vi "高低位调试.vi"() -> ()   [LabVIEW 2016]
uses:
  <vilib>/Plasmionique/MB Master/MB_Master_Serial/MB_Master_Serial.lvclass
  C:/Program Files (x86)/National Instruments/LabVIEW 2016/vi.lib/Plasmionique/MB Master/MB_Master/MB_Master.lvclass
  <vilib>/Plasmionique/MB Master/MB Master.lvlib
panel:
  out "data":u16[](array[numeric]) format="%04xH"
  out "测量数据区":T1
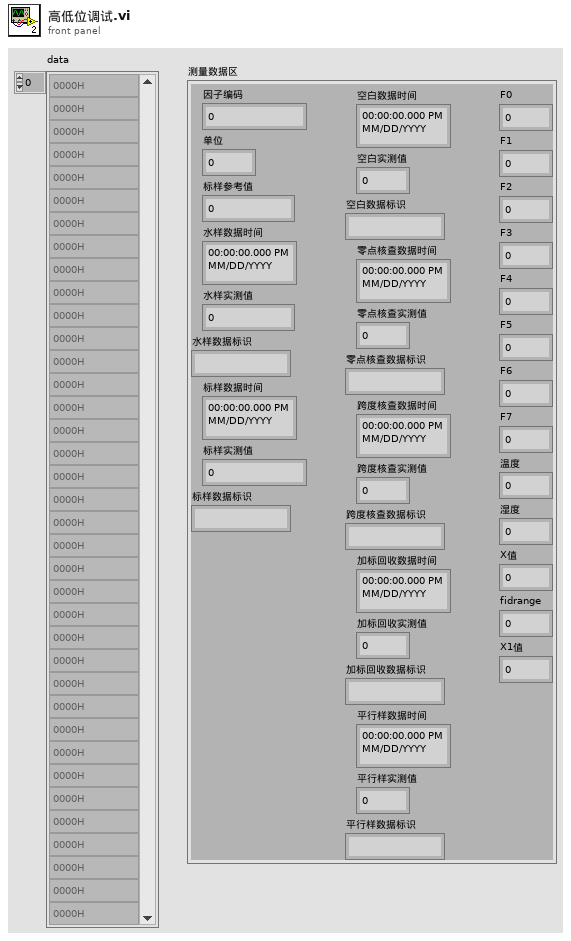
[diagram p1: front panel]
types:
  T1 = cluster{"因子编码":u32, "单位":u16, "标样参考值":sgl, "水样数据时间":timestamp, "水样实测值":sgl, "水样数据标识":string, "标样数据时间":timestamp, "标样实测值":sgl, "标样数据标识":string, "空白数据时间":timestamp, "空白实测值":sgl, "空白数据标识":string, "零点核查数据时间":timestamp, "零点核查实测值":sgl, "零点核查数据标识":string, "跨度核查数据时间":timestamp, "跨度核查实测值":sgl, "跨度核查数据标识":string, "加标回收数据时间":timestamp, "加标回收实测值":sgl, "加标回收数据标识":string, "平行样数据时间":timestamp, "平行样实测值":sgl, "平行样数据标识":string, "F0":sgl, "F1":sgl, "F2":sgl, "F3":sgl, "F4":sgl, "F5":sgl, "F6":sgl, "F7":sgl, "温度":sgl, "湿度":sgl, "X值":sgl, "fidrange":u16, "X1值":sgl}
  T2 = cluster{"baud rate (bps)":u32, "stop bits":u16, "parity":u16, "flow control":u16, "timeout":u32, "retries":i32}
  T3 = cluster{"因子编码":u32, "单位":u16, "标样参考值":sgl, "水样数据时间":timestamp, "水样实测值":sgl, "水样数据标识":string, "标样数据时间":timestamp, "标样实测值":sgl, "标样数据标识":string, "空白数据时间":timestamp, "空白实测值":sgl, "空白数据标识":string, "零点核查数据时间":timestamp, "零点核查实测值":sgl, "零点核查数据标识":string, "跨度核查数据时间":timestamp, "跨度核查实测值":sgl, "跨度核查数据标识":string, "加标回收数据时间":timestamp, "加标回收实测值":sgl, "加标回收数据标识":string, "平行样数据时间":timestamp, "平行样实测值":sgl, "平行样数据标识":string, "F0":sgl, "F1":sgl, "F2":sgl, "F3":sgl, "F4":sgl, "F5":sgl, "F6":sgl, "F7":sgl, "温度":sgl, "湿度":sgl, "X值":sgl, "fidrange":u16, "X1值":sgl}[]
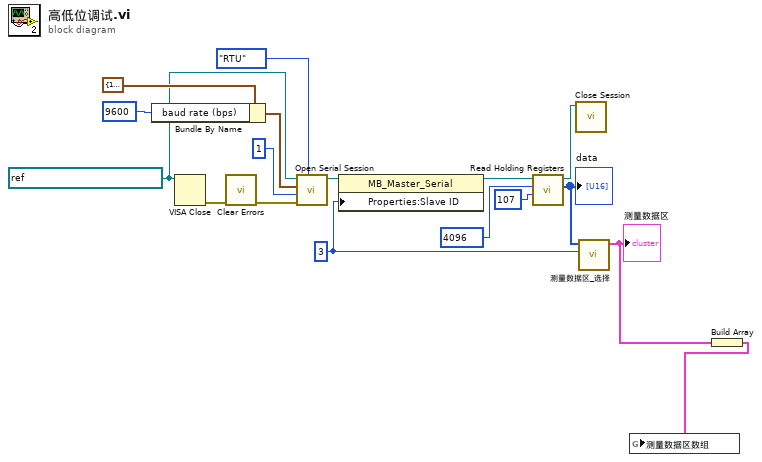
[diagram p0: block diagram]
diagram:
  w6 = refnum<visa-resource-name> "COM7" ("VISA Resource")
  w8 = u8 3 ("Slave ID")
  n1 = Bundle By Name(cluster=T2 {"baud rate (bps)"=115200, "stop bits"=10, "parity"=0, "flow control"=0, "timeout"=1000, "retries"=1} ("Serial Config"), "baud rate (bps)"=u32 9600) -> (w14:T2)
  n2 = VISA Close(VISA resource name=w6) -> (error out=w3:errorcluster)  [unwired: 1 in]
  n3 = call <vilib>:"Clear Errors.vi"("error in (no error)"=w3) -> ("error out"=w13:errorcluster)  [unwired: 5 in, 1 out]
  n4 = call <vilib>:"Open Serial Session.vi"("Mode (RTU)"=enum16{"RTU", "ASCII"}."RTU", "Error in"=w13, "Slave ID"=u8 1, "Serial Config"=w14, "VISA Resource"=w6) -> ("MB_Serial session"=w9:refnum<class "MB_Master_Serial.lvclass">)  [unwired: 5 in, 1 out]
  n5 = property class="MB_Master_Serial"(reference=w9, "Properties:Slave ID"=w8) -> (reference out=w11:refnum<class "MB_Master_Serial.lvclass">)  [unwired: 1 in, 1 out]
  n6 = call <vilib>:"Read Holding Registers.vi"("quantity"=u16 107, "starting address"=u16 4096, "MB session in"=w11) -> ("Registers"=w7:u16[], "MB session out"=w4:refnum<class "MB_Master_Serial.lvclass">)  [unwired: 6 in, 1 out]
  "data" <- w7
  n7 = call-dynamic "Close Session.vi"("MB_Serial session"=w4) -> ()  [unwired: 10 in, 1 out]
  n8 = call "测量数据区_选择.vi"("Slave ID"=w8, "data"=w7) -> ("测量数据区"=w2:T1)  [unwired: 9 in]
  "测量数据区" <- w2
  n9 = Build Array(w2) -> (w1:T3)
  n10 = global write "VAR总磷总氮全局变量.vi" "测量数据区数组"(w1) -> ()
